vi "Backlight Command.vi"(8 "error in (no error)":errorcluster, 10 "ON/OFF":bool, 11 "VISA resource name":refnum<visa-resource-name>) -> (0 "error out":errorcluster, 3 "VISA resource name out":refnum<visa-resource-name>)   [LabVIEW 2015, in "Keysight U1252.lvlib"]
doc: "VI used turn on and turn off multimeter backlight."
uses:
  <instrlib>/Keysight U1252/Keysight U1252.lvlib
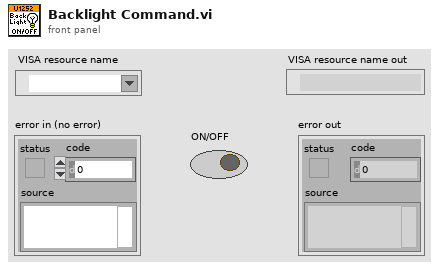
[diagram p1: front panel]
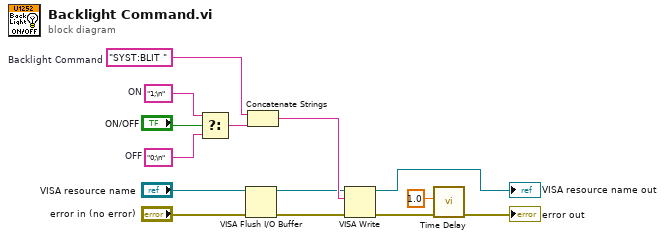
[diagram p0: block diagram]
diagram:
  w8 = "0;\n"  # OFF
  w10 = "1;\n"  # ON
  w6 = "SYST:BLIT "  # Backlight Command
  n1 = Select(t=w10, s="ON/OFF", f=w8) -> (s? t:f=w7:string)
  n2 = VISA Flush I/O Buffer(VISA resource name="VISA resource name", error in (no error)="error in (no error)") -> (VISA resource name out=w2:refnum<visa-resource-name>, error out=w1:errorcluster)  [unwired: 1 in]
  n3 = Concatenate Strings(w6, w7) -> (w5:string)
  n4 = VISA Write(VISA resource name=w2, write buffer=w5, error in (no error)=w1) -> (VISA resource name out=→"VISA resource name out":refnum<visa-resource-name>, error out=w14:errorcluster)  [unwired: 1 out]
  n5 = call "Time Delay"("error in (no error)"=w14, "Delay Time (s)"=1.0) -> ("error out"=→"error out":errorcluster)  [unwired: 9 in]
